vi "Scanner.vi"(4 "Blue or Luma or Val or Inten Range":cluster{"Lower value":i32, "Upper value":i32}={"Lower value"=0, "Upper value"=255}, 6 "Green or Sat Range":cluster{"Lower value":i32, "Upper value":i32}={"Lower value"=0, "Upper value"=255}, 8 "error in (no error)":errorcluster, 9 "Image Dst":T1, 10 "Image Src":T1, 11 "Red or Hue Range":cluster{"Lower value":i32, "Upper value":i32}={"Lower value"=0, "Upper value"=255}) -> (0 "error out":errorcluster)   [LabVIEW 2019]
uses:
  <vilib>/vision/Image Controls.llb/IMAQ Image.ctl
  <vilib>/vision/NI_Vision_Development_Module.lvlib
panel:
  out "Centroid":cluster{"X Centroid":sgl, "Y Centroid":sgl} {"Y Centroid" format="%.2f"; "X Centroid" format="%.2f"}
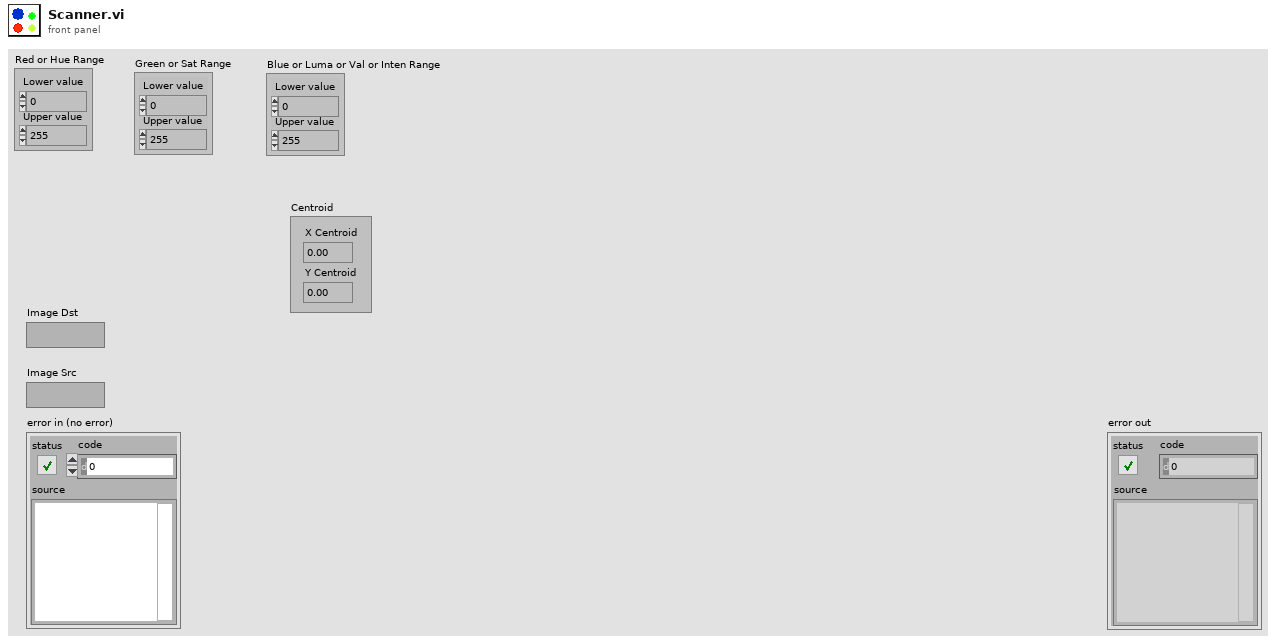
[diagram p1: front panel]
types:
  T1 = typedef "IMAQ Image.ctl" = refnum<image>
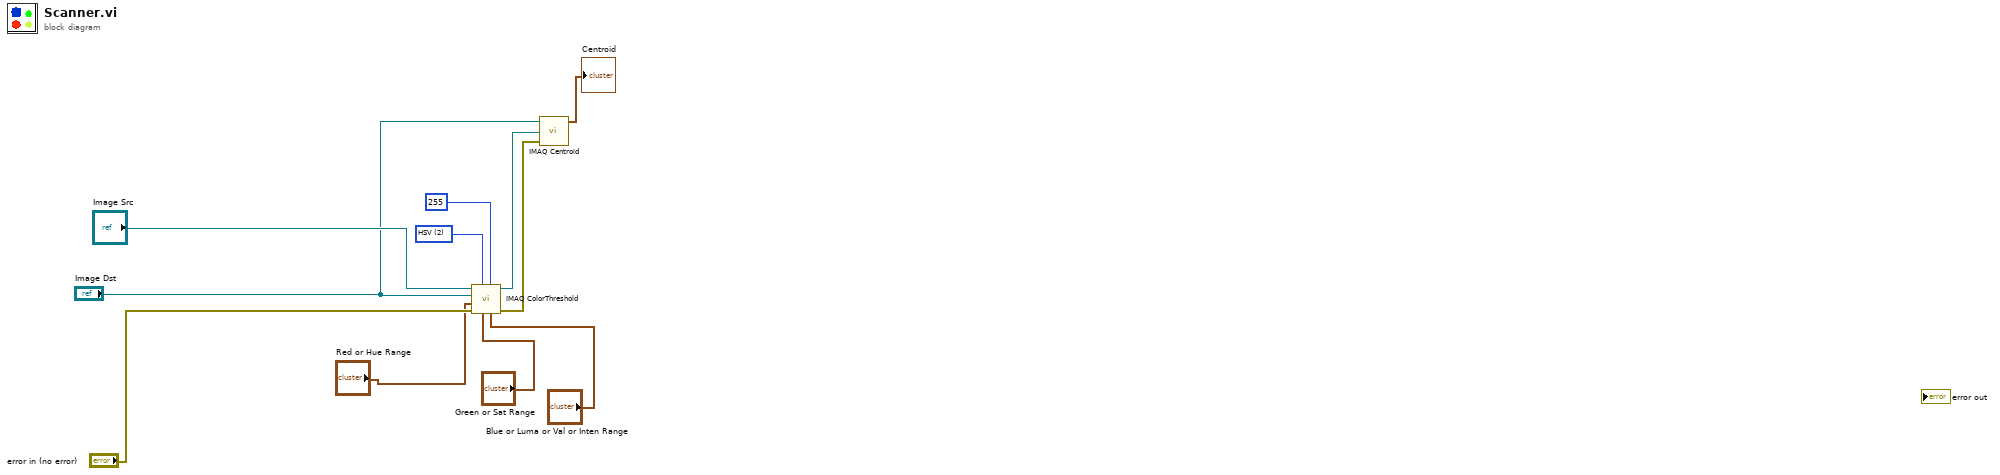
[diagram p0: block diagram]
diagram:
  w10 = u16 2 items=["RGB", "HSL", "HSV", "HSI"] ("Color Mode")
  n1 = call "IMAQ ColorThreshold"("Blue or Luma or Val or Inten Range"="Blue or Luma or Val or Inten Range", "Replace Value"=255, "Green or Sat Range"="Green or Sat Range", "Color Mode"=w10, "error in (no error)"="error in (no error)", "Red or Hue Range"="Red or Hue Range", "Image Dst"="Image Dst", "Image Src"="Image Src") -> ("error out"=w8:errorcluster, "Image Dst Out"=w9:T1)  [unwired: 2 in]
  n2 = call "IMAQ Centroid"("error in (no error)"=w8, "Image Mask"=w9, "Image"="Image Dst") -> ("Centroid"=→"Centroid":cluster{"X Centroid":sgl, "Y Centroid":sgl})  [unwired: 1 in, 1 out]
